vi "Close.vi"(8 "Error In":errorcluster, 11 "Keithley 7001 In":refnum<visa-resource-name>) -> (0 "Error Out":errorcluster)   [LabVIEW 2012, in "Keithley-7001.lvlib"]
uses:
  Keithley-7001.lvlib
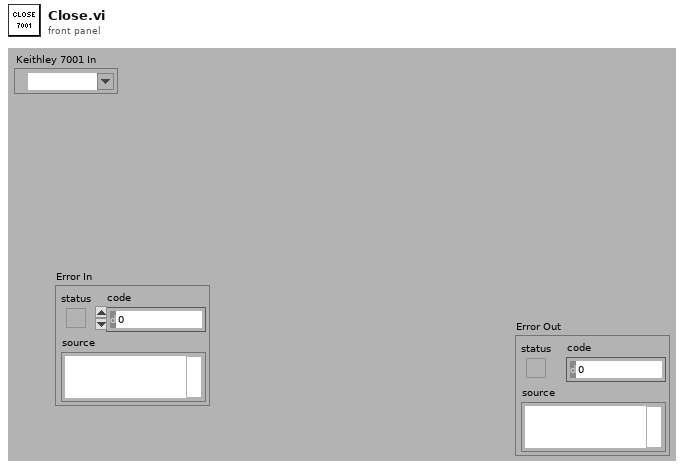
[diagram p1: front panel]
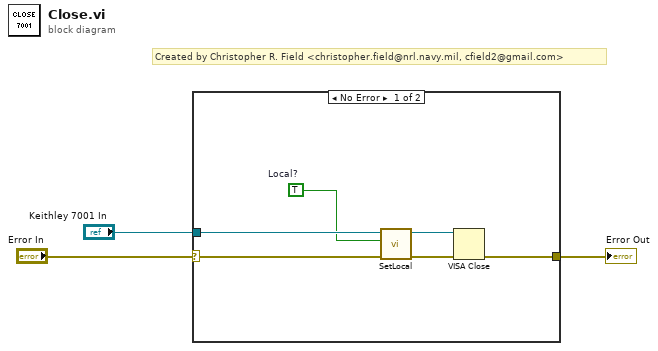
[diagram p0: block diagram]
diagram:
  # "Created by Christopher R. Field <christopher.field@nrl.navy.mil, cfield2@gmail.com>"
  n1 = case shown="No Error" "Error In" {
    selector: "Error In" -> [w4 w10]
    tunnel: [w9 w10] -> w3
    tunnel: "Keithley 7001 In" -> [w8 _]
    frame No Error {
      w7 = TRUE  # Local?
      n2 = call "SetLocal.vi"("Error In"=w4, "Local?"=w7, "Keithley 7001 In"=w8) -> ("Error Out"=w5:errorcluster, "Keithley 7001 Out"=w6:refnum<visa-resource-name>)  [unwired: 7 in]
      n3 = VISA Close(VISA resource name=w6, error in (no error)=w5) -> (error out=w9:errorcluster)
    }
    frame Error {
    }
  }
  "Error Out" <- w3
